vi "SCM10_GET_TEMP.vi"(8 "ERR IN":errorcluster, 11 "I/O IN":T1={"I/O Select (Serial: 0)"=enum."Serial", "VISA"="ASRL0::INSTR", "IP Address"="192.168.111.127", "Baud Rate"=enum."115200", "COM"=1}) -> (0 "ERR OUT":errorcluster, 2 "Temperature (K)":dbl, 3 "I/O OUT":T1={"I/O Select (Serial: 0)"=enum."Serial", "VISA"="COM1", "IP Address"="192.168.111.127", "Baud Rate"=enum."19200", "COM"=1})   [LabVIEW 2016]
panel:
  # "Temperature (K)"
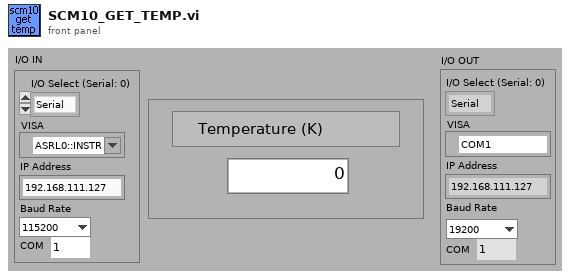
[diagram p1: front panel]
types:
  T1 = cluster{"I/O Select (Serial: 0)":enum16{"Serial", "TCP"}, "VISA":refnum<visa-resource-name>, "IP Address":string, "Baud Rate":enum16{"9600", "19200", "57600", "115200"}, "COM":i32}
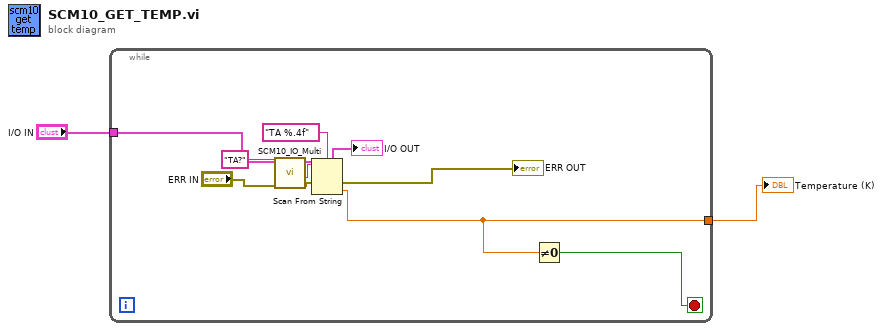
[diagram p0: block diagram]
diagram:
  n1 = while {
    tunnel: [w4] -> w2
    tunnel: "I/O IN" -> [w3]
    stop <- w5 stop-if-true
    n2 = call "SCM10_IO_Multi.vi"("ERR IN"="ERR IN", "QUERY"="TA?", "I/O IN"=w3) -> ("ERR OUT"=w9:errorcluster, "RESPONSE"=w6:string, "I/O OUT"=→"I/O OUT":T1)  [unwired: 1 in, 1 out]
    n3 = Scan From String(format string="TA %.4f", input string=w6, error in=w9) -> (error out=→"ERR OUT":errorcluster, output 1=w4:dbl)  [unwired: 2 in, 2 out]
    n4 = Not Equal To 0?(x=w4) -> (x != 0?=w5:bool)
  }
  "Temperature (K)" <- w2
